vi "PIDparallelController.vi"(0 "Proportional Gain":dbl=1.0, 1 "Integral Gain":dbl=1.0, 2 "Error IN":dbl, 4 "High Frequency [s] (Tf)":dbl=1.0, 5 "Derivative Gain":dbl=1.0) -> (7 "Controller Output":dbl)   [LabVIEW 2012]
uses:
  <vilib>/Simulation/Model Libraries/PID/subVIs/SIM PID Derivative Gain.vi
  <vilib>/Simulation/Model Libraries/PID/subVIs/SIM PID Integral Gain.vi
  <vilib>/Simulation/Implementation/Shared/SIMSCR Execution Mode.ctl
  <vilib>/Simulation/Scripting/Companion Diagram/SimConfigNode/SimParams.ctl
  <vilib>/Simulation/Scripting/Companion Diagram/SimConfigNode/_simSolvers.ctl
  <vilib>/Simulation/Param Hierarchy/Typedefs/SIMPH Param Control Actions.ctl
  <vilib>/Simulation/Implementation/Shared/NILVSim_ParamChanged.vi
  <vilib>/Simulation/SignalArithmetic/Implementation/NILVSim Gain.llb/SIM Gain (scalar).vi
  <vilib>/Simulation/Implementation/Shared/NILVSim_Manager.vi
  <vilib>/Simulation/Implementation/Shared/NILVSim_FinalizeModel.vi
  <vilib>/Simulation/Implementation/Shared/SIM Unbundle Sim Info.vi
  <vilib>/Utility/error.llb/Clear Errors.vi
  <vilib>/Simulation/Implementation/Shared/NILVSim_GetModelError.vi
  <vilib>/Simulation/Implementation/Shared/SIM SimErrorHandler.vi
  <vilib>/Simulation/Implementation/Shared/SIM Bundle Sim Info.vi
  <vilib>/Simulation/Implementation/Shared/NILVSim_Initialize.vi
  <vilib>/Simulation/Utility/Implementation/NILVSim Get Time and IsAcceptedStep.vi
  <vilib>/Simulation/Implementation/Shared/SIMSH Read Queue.vi
  <vilib>/Simulation/Scripting/Companion Diagram/SimConfigNode/SimDog.xnode
  <vilib>/Simulation/Implementation/XNodeFramework/SimXNode/SimX.xnode
  <vilib>/Simulation/Implementation/Shared/NI_SIM_Implementation.lvlib
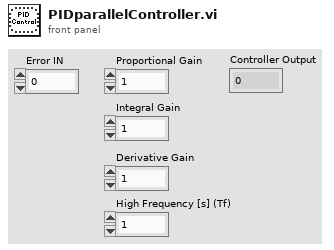
[diagram p1: front panel]
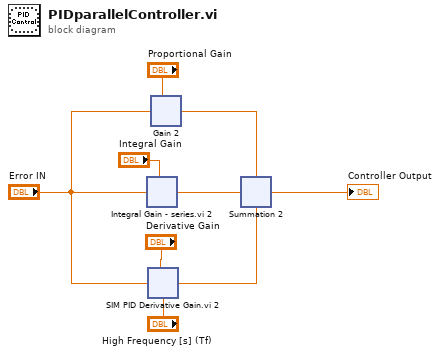
[diagram p0: block diagram]
diagram:
  n1 = xnode ("Integral Gain - series.vi 2")("Integral Gain"="Integral Gain", "Error"="Error IN") -> ("output"=w8:dbl)  [unwired: 2 in, 11 out]
  n2 = xnode ("SIM PID Derivative Gain.vi 2")("Derivative Gain"="Derivative Gain", "Error"="Error IN", "High Frequency [s] (Tf)"="High Frequency [s] (Tf)") -> ("output"=w4:dbl)  [unwired: 12 out]
  n3 = xnode ("Gain 2")("gain"="Proportional Gain", "input"="Error IN") -> ("output"=w3:dbl)  [unwired: 2 in]
  n4 = xnode ("Summation 2")("Operand1"=w3, "Operand2"=w8, "Operand3"=w4) -> ("Result"=→"Controller Output":dbl)
